vi "Set Virt Instr CFG.vi"(8 "error in":errorcluster, 10 "Virt Instr CFG":string, 11 "Configuration UI Actor in":refnum<class "Configuration UI Actor.lvclass">) -> (0 "error out":errorcluster, 3 "Configuration UI Actor out":refnum<class "Configuration UI Actor.lvclass">)   [LabVIEW 2023, in "Configuration UI Actor.lvlib" / "Configuration UI Actor.lvclass"]
uses:
  Configuration UI Actor.lvclass
  Configuration UI Actor.lvclass/Configuration UI Actor.ctl
  <vilib>/JDP Science/JSONtext/JSONtext.lvlib
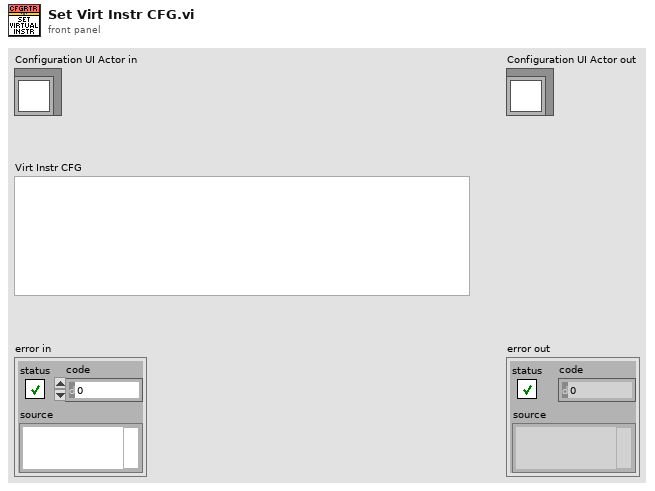
[diagram p1: front panel]
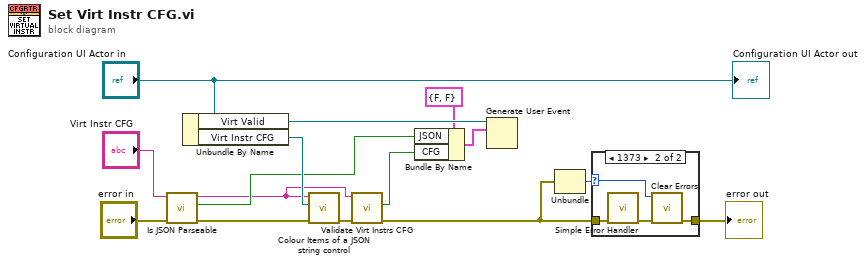
[diagram p0: block diagram]
diagram:
  n1 = call "Is JSON Parseable.vi"("error in"="error in", "<JSON>"="Virt Instr CFG") -> ("error out"=w11:errorcluster, "Valid?"=w7:bool, "Pretty <JSON>"=w5:string)  [unwired: 7 in]
  n2 = Unbundle By Name("Configuration UI Actor in") -> ("Virt Valid"=w10:refnum<user-event>, "Virt Instr CFG"=w14:refnum<vi>)
  n3 = call <vilib>:"Colour Items of a JSON string control.vi"("error in (no error)"=w11, "String Control"=w14, "JSON"=w5) -> ("error out"=w6:errorcluster)  [unwired: 8 in]
  n4 = call "Validate Virt Instrs CFG.vi"("error in"=w6, "<JSON>"=w5) -> ("error out"=w1:errorcluster, "Is Valid?"=w4:bool)  [unwired: 8 in]
  n5 = Bundle By Name(cluster=cluster{"JSON":bool, "CFG":bool} {"JSON"=FALSE, "CFG"=FALSE} ("Virt Valid"), "JSON"=w7, "CFG"=w4) -> (w8:cluster{"JSON":bool, "CFG":bool})
  n6 = Generate User Event(user event=w10, event data cluster=w8) -> ()  [unwired: 2 in, 2 out]
  n7 = Unbundle(w1) -> ("code"=w2:i32)  [unwired: 2 out]
  n8 = case shown="1373" w2 {
    selector: w2 -> [_ w18]
    tunnel: w1 -> [w16 w20]
    tunnel: [w16 w19] -> w3
    frame Default {
    }
    frame 1373 {
      n9 = call <vilib>:"Simple Error Handler.vi"("error in (no error)"=w20) -> ("error out"=w17:errorcluster)  [unwired: 4 in, 4 out]
      n10 = call <vilib>:"Clear Errors.vi"("error in (no error)"=w17, "specific error code to clear (0: all)"=w18) -> ("error out"=w19:errorcluster)  [unwired: 4 in, 1 out]
    }
  }
  "error out" <- w3
  "Configuration UI Actor out" <- "Configuration UI Actor in"
